vi "zero_continuos.vi"(11 "StrainGauges":cluster{"Array":timestamp[], "Data":dbl[]}[](array[cluster])) -> (3 "StrainGauges out":cluster{"Array":timestamp[], "Array":dbl[]}[](array[cluster]))   [LabVIEW 2016]
uses:
  <vilib>/Analysis/baseanly.llb/Mean (DBL).vi
  <vilib>/Analysis/NI_AALBase.lvlib
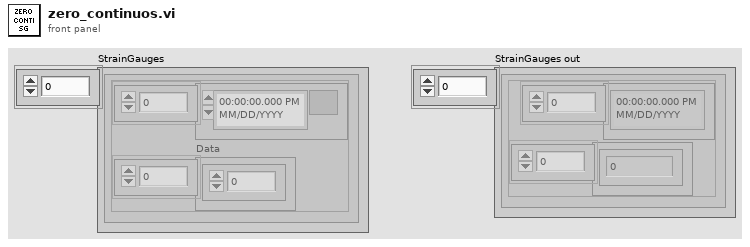
[diagram p1: front panel]
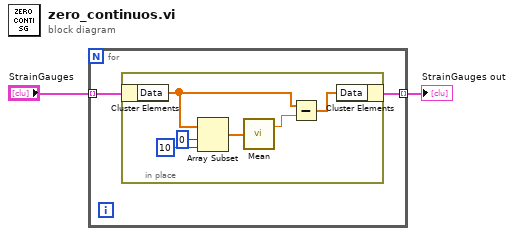
[diagram p0: block diagram]
diagram:
  n1 = for {
    tunnel: "StrainGauges" -> [w4] mode=indexing
    tunnel: [w3] -> w1 mode=indexing
    n2 = in-place {
      n3 = in-place-cluster #1(w4) -> ("Data"=w6:dbl[])
      n4 = Array Subset(array=w6, index=0, length=10) -> (w8:dbl[])
      n5 = call-poly <vilib>:"Mean.vi"("X"=w8) -> ("mean"=w7:dbl)  [unwired: 1 out]
      n6 = Subtract(x=w6, y=w7) -> (x-y=w5:dbl[])
      n7 = in-place-cluster #1("Data"=w5) -> (w3:cluster{"Array":timestamp[], "Data":dbl[]})
    }
  }
  "StrainGauges out" <- w1
